vi "Get Destinations In Use.vi"(8 "error in (no error)":errorcluster, 11 "SigMan in":refnum<class "SignalManager.lvclass">) -> (0 "error out":errorcluster, 2 "Destinations in use":string[](array[string]), 3 "SigMan out":refnum<class "SignalManager.lvclass">)   [LabVIEW 2015, in "SignalManager.lvclass"]
uses:
  SignalManager.lvclass
  SignalManager.lvclass/SignalManager.ctl
  Channel/Channel.lvclass/Channel.ctl
  Channel/Read Destination.vi
  Channel/Channel.lvclass
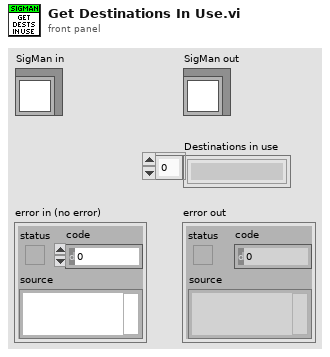
[diagram p1: front panel]
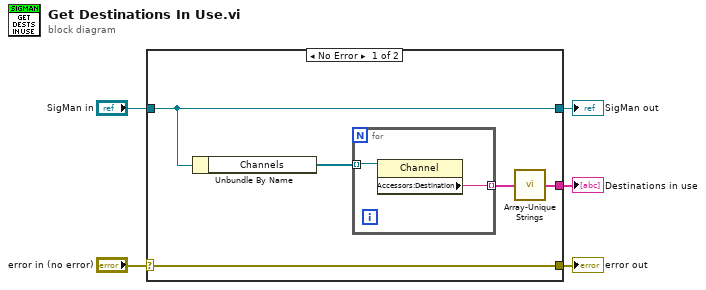
[diagram p0: block diagram]
diagram:
  n1 = case shown="No Error" "error in (no error)" {
    selector: "error in (no error)" -> [w10 w14]
    tunnel: [w10 w14] -> w4
    tunnel: [w8 w13] -> w2
    tunnel: "SigMan in" -> [w8 w13]
    tunnel: [w6 _] -> w1
    frame No Error {
      n2 = Unbundle By Name(w8) -> ("Channels"=w9:refnum<class "Channel.lvclass">[])
      n3 = for {
        tunnel: w9 -> [w12] mode=indexing
        tunnel: [w11] -> w7 mode=indexing
        n4 = property class="Channel"(reference=w12) -> ("Accessors:Destination"=w11:string)  [unwired: 1 in, 2 out]
      }
      n5 = call "Array-Unique Strings.vi"("Strings"=w7) -> ("Unique strings"=w6:string[])  [unwired: 4 in]
    }
    frame Error {
    }
  }
  "error out" <- w4
  "SigMan out" <- w2
  "Destinations in use" <- w1
